vi "test_integration.vi"() -> ()   [LabVIEW 2018]
uses:
  <vilib>/addons/Modulation/Digital/Channel Coding/MT Convolutional Encoder (Rate).vi
  <vilib>/addons/Modulation/Digital/Support/Common/Validators/mod_Validate Bit Stream.vi
  <vilib>/addons/Modulation/Digital/Channel Coding/Convolutional codes/mod_Convolutional encoder.vi
  <vilib>/addons/Modulation/Analog/support/mod_Set Error Source.vi
  <vilib>/addons/Modulation/Digital/Channel Coding/Convolutional codes/subVIs/mod_Generate encoder tap connections.vi
  <vilib>/addons/Modulation/Digital/Channel Coding/Convolutional codes/subVIs/mod_Perform convolutional encoding.vi
  <vilib>/addons/Modulation/Digital/Channel Coding/Block codes/subVIs/mod_Buffer block code info (I8).vi
  <vilib>/addons/Modulation/Digital/Channel Coding/Convolutional codes/subVIs/mod_Generate valid reset (convolutional, I8).vi
  <vilib>/addons/Modulation/Digital/Channel Coding/Convolutional codes/subVIs/mod_Select known generator matrix.vi
  <vilib>/addons/Modulation/Digital/Support/Common/Validators/mod_Validate Convolutional Encoder prms.vi
  <vilib>/addons/Modulation/niDMT.lvlib
panel:
  out "input bits":i8[](array[numeric])
  out "built-in encoder stream":i8[](array[numeric])
  out "personnal encoder stream":i8[](array[numeric])
  in  "Rate (k/n)":enum16{"1/2", "1/3", "1/4", "2/3", "3/4"}(ring)
  in  "k":i32
  out "sortie générateur":string
  out "sortie codeur convolutif":string
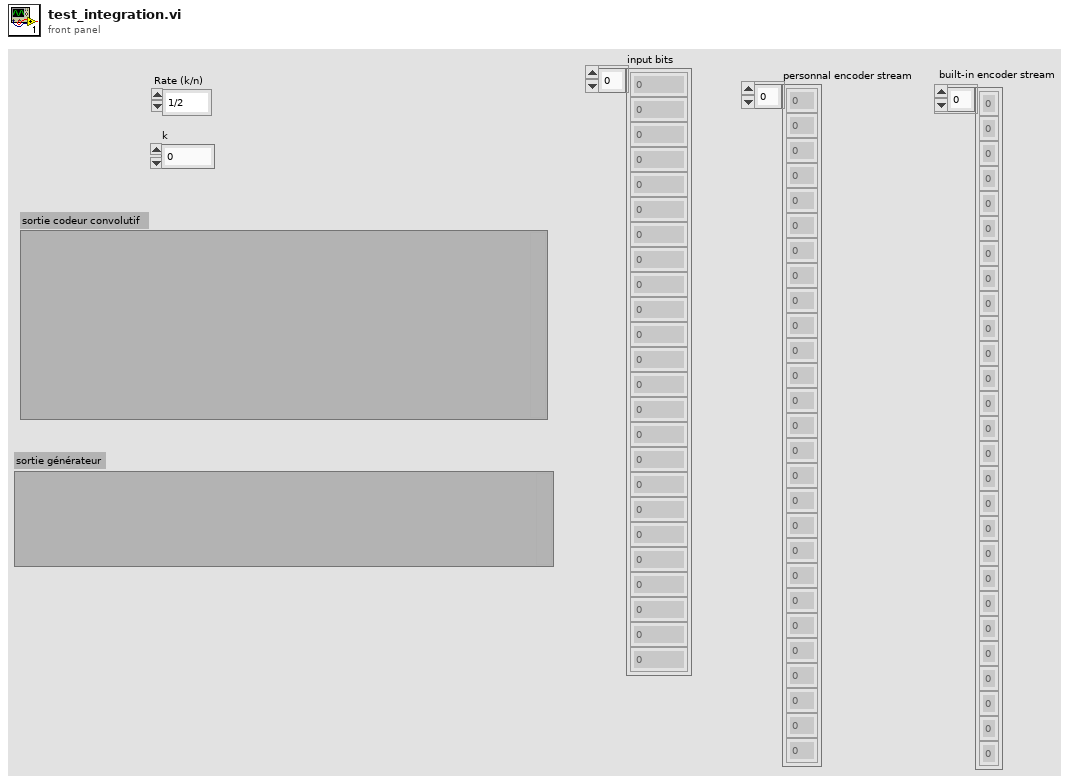
[diagram p1: front panel]
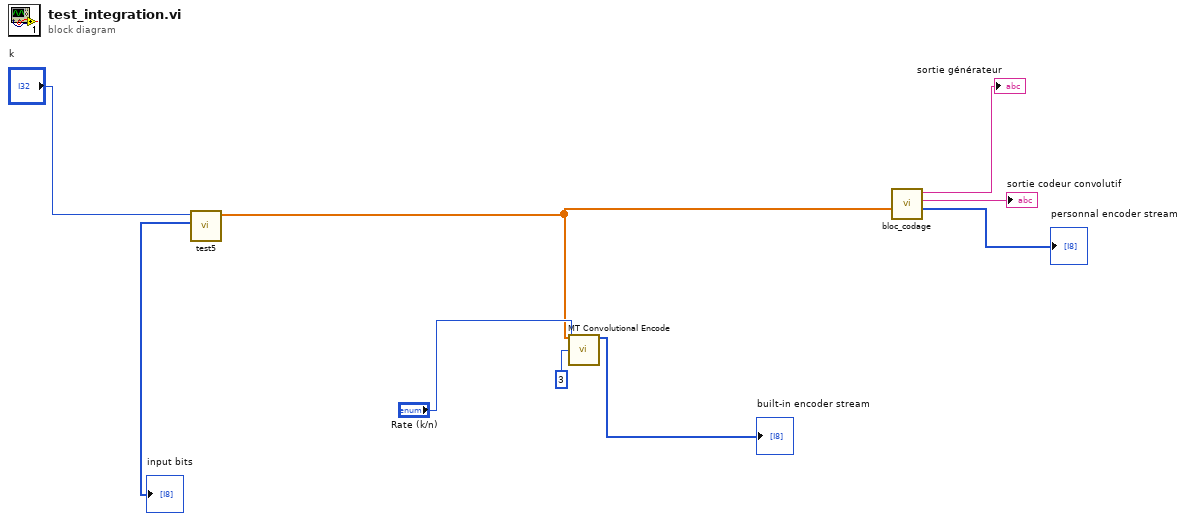
[diagram p0: block diagram]
diagram:
  n1 = call "test5.vi"("k"="k") -> ("output bit stream"=→"input bits":i8[], "Array"=w2:dbl[])  [unwired: 9 in]
  n2 = call-poly <vilib>:"MT Convolutional Encode.vi"("input bit stream"=w2, "rate (k/n)"="Rate (k/n)", "constraint length (K)"=3) -> ("output bit stream"=→"built-in encoder stream":i8[])  [unwired: 10 in, 2 out]
  n3 = call "bloc_codage.vi"("Array in"=w2) -> ("output bit stream"=→"personnal encoder stream":i8[], "sortie codeur convolutif"=→"sortie codeur convolutif":string, "sortie générateur"=→"sortie générateur":string)  [unwired: 8 in]
